vi "LoadController.vi"(8 "error in (no error)":errorcluster, 10 "Actor In":refnum<class "Actor.lvclass">, 11 "Stage_MadCityLab in":refnum<class "Stage_MadCityLab.lvclass">) -> (0 "error out":errorcluster, 3 "Stage_MadCityLab out":refnum<class "Stage_MadCityLab.lvclass">)   [LabVIEW 2020, in "Stage_MadCityLab.lvlib" / "Stage_MadCityLab.lvclass"]
uses:
  Stage_MadCityLab.lvclass
  ViewController/TripleAxisStageController/TriaxesStageController.lvclass
  Hardware Abstraction Layer/Component/Stage/Stage/Stage.lvclass
  C:/Program Files/National Instruments/LabVIEW 2020/vi.lib/ActorFramework/Actor/Actor.lvclass
  <vilib>/ActorFramework/Actor/Actor.lvclass
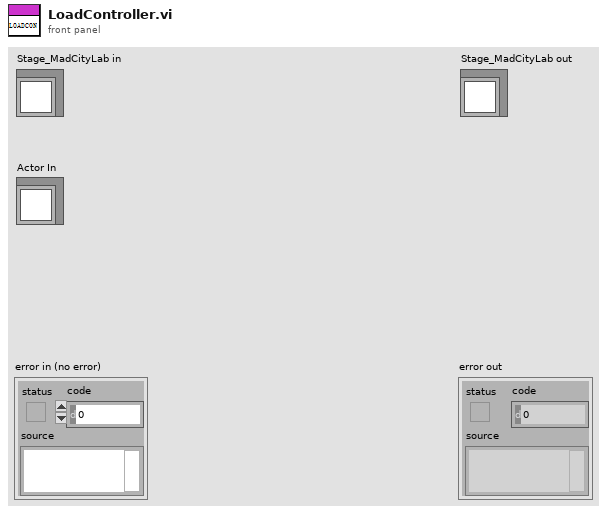
[diagram p1: front panel]
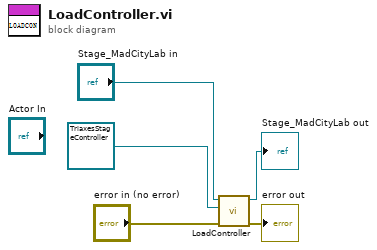
[diagram p0: block diagram]
diagram:
  n1 = call-parent "LoadController.vi"("error in (no error)"="error in (no error)", "Actor In"=refnum<class "TriaxesStageController.lvclass"> refnum ("TripleAxisStageController.lvlib:TripleAxisStageController.lvclass"), "Device in"="Stage_MadCityLab in") -> ("error out"=→"error out":errorcluster, "Device out"=→"Stage_MadCityLab out":refnum<class "Stage_MadCityLab.lvclass">)  [unwired: 7 in]
